vi "BotSpeakSerial_WriteRead1.vi"(4 "To Write":string, 5 "error In":errorcluster, 6 "Timeout":i32, 7 "Retries":i8, 8 "Address":string) -> (0 "error out":errorcluster, 1 "Reply":string, 2 "Reply EOF":string)   [LabVIEW 2012]
uses:
  <userlib>/botspeak/VIs/SubVIs/BotSpeak_Globals.vi
panel:
  out "iterations":i32
  out "Buffer":u32[](graph)
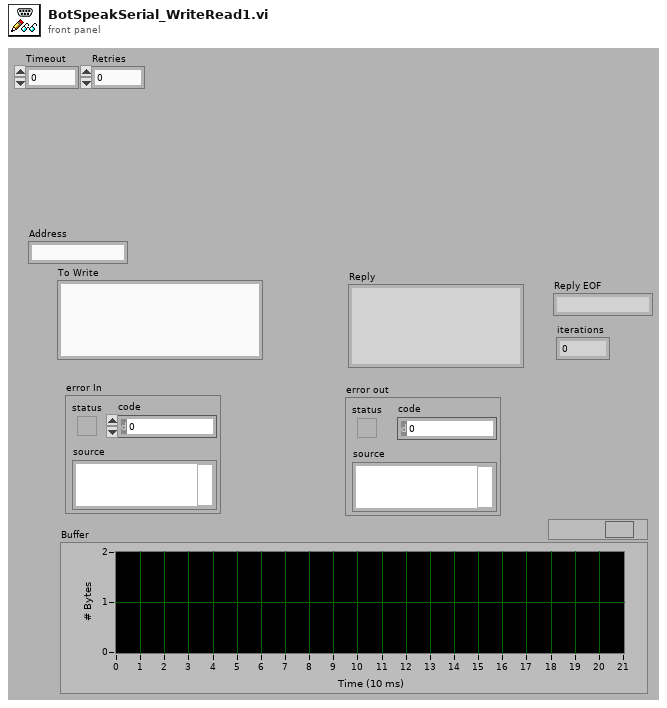
[diagram p1: front panel]
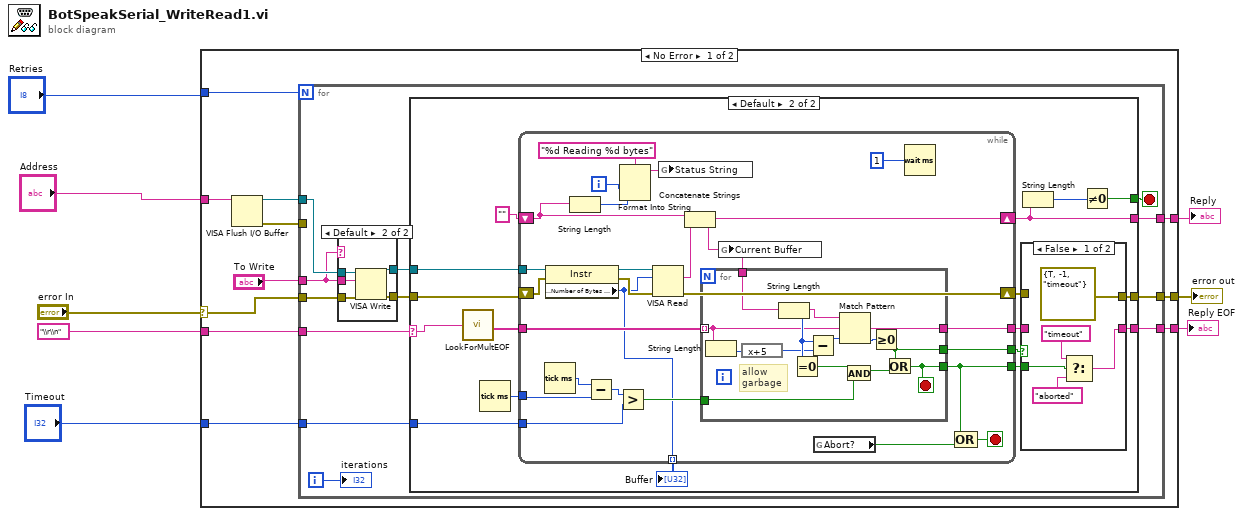
[diagram p0: block diagram]
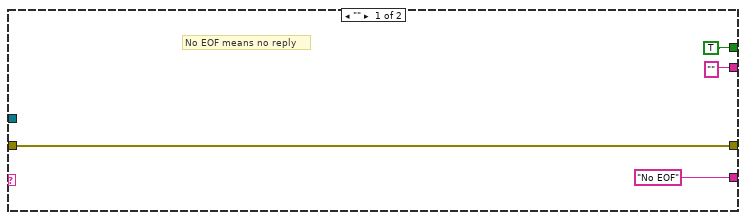
[diagram p3: hidden frame]
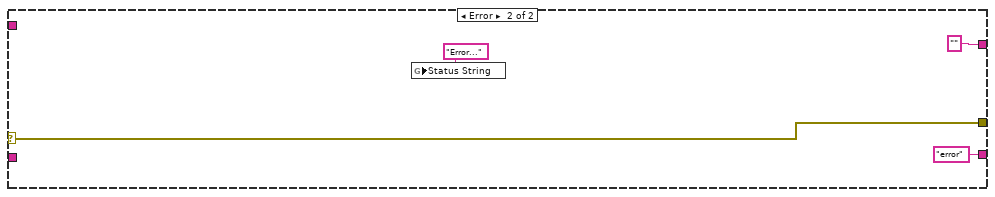
[diagram p5: hidden frame]
diagram:
  n1 = case shown="No Error" "error In" {
    selector: "error In" -> [w13 w105]
    tunnel: [w19 ""] -> w6
    tunnel: [w18 w105] -> w7
    tunnel: "Retries" -> [w17 _]
    tunnel: "Address" -> [w11 _]
    tunnel: "Timeout" -> [w16 _]
    tunnel: "\\r\\n" ("Reply EOF") -> [w14 _]
    tunnel: [w12 "error" ("Reply EOF")] -> w5
    frame No Error {
      n2 = VISA Flush I/O Buffer(VISA resource name=w11) -> (VISA resource name out=w9:refnum<visa-resource-name>, error out=w10:errorcluster)  [unwired: 2 in]
      n3 = for {
        N: w17 -> [_]
        tunnel: "To Write" -> [w21]
        tunnel: [w31] -> w19
        tunnel: [w27] -> w18
        tunnel: w13 -> [w30]
        tunnel: w16 -> [w25]
        tunnel: w14 -> [w24]
        tunnel: w9 -> [w23]
        tunnel: [w22] -> w12
        tunnel: w10 -> [_]
        i -> [w20]
        stop <- w26 stop-if-true
        n4 = case shown="Default" w21 {
          tunnel: w21 -> [_ w38]
          tunnel: w30 -> [w33 w37]
          tunnel: [w32 w36] -> w29
          tunnel: [w33 w35] -> w28
          tunnel: w23 -> [w32 w34]
          frame "" {
          }
          frame Default {
            n5 = VISA Write(VISA resource name=w34, write buffer=w38, error in (no error)=w37) -> (VISA resource name out=w36:refnum<visa-resource-name>, error out=w35:errorcluster)  [unwired: 1 out]
          }
        }
        n6 = case shown="Default" w24 {
          selector: w24 -> [_ w45]
          tunnel: ["" w55] -> w31
          tunnel: [w41 w44] -> w27
          tunnel: w29 -> [_ w58]
          tunnel: w28 -> [w41 w57]
          tunnel: [TRUE w47] -> w26
          tunnel: w25 -> [_ w53]
          tunnel: ["No EOF" ("Reply EOF") w49] -> w22
          frame "" {
            # "No EOF means no reply"
          }
          frame Default {
            n7 = call <userlib>:"LookForMultEOF.vi"("Reply EOF"=w45) -> ("Array"=w52:string[])
            n8 = Tick Count (ms)() -> (millisecond timer value=w56:u32)
            n9 = while {
              tunnel: w52 -> [w86]
              shift-right: [w91] -> w43
              shift-left: w57 -> [w90]
              shift-right: [w73] -> w55
              shift-left: "" -> [w76]
              tunnel: w58 -> [w85]
              tunnel: w56 -> [w80]
              tunnel: w53 -> [w71]
              tunnel: [w69] -> w51
              tunnel: [w70] -> w50
              tunnel: [w68] -> w48
              tunnel: [w67] -> w46 mode=indexing
              i -> [w78]
              stop <- w82 stop-if-true
              n10 = Tick Count (ms)() -> (millisecond timer value=w81:u32)
              n11 = property class="Instr"(reference=w85, error in=w90) -> (reference out=w89:refnum<visa-resource-name>, error out=w88:errorcluster, "Serial Settings:Number of Bytes at Serial Port"=w67:u32)
              n12 = String Length(string=w76) -> (length=w75:i32)
              n13 = Subtract(x=w81, y=w80) -> (x-y=w84:u32)
              n14 = Greater?(x=w84, y=w71) -> (0:w83:bool)
              n15 = Format Into String(format string="%d Reading %d bytes", w78, w75) -> (resulting string=w77:string)  [unwired: 2 in, 1 out]
              n16 = VISA Read(VISA resource name=w89, byte count=w67, error in (no error)=w88) -> (read buffer=w87:string, error out=w91:errorcluster)  [unwired: 2 out]
              n17 = global write "BotSpeak_Globals.vi" "Status String"(w77) -> ()
              n18 = Concatenate Strings(w76, w87) -> (w73:string)
              n19 = for {
                tunnel: w86 -> [w95] mode=indexing
                tunnel: w83 -> [w102]
                tunnel: w73 -> [w93]
                tunnel: [w96] -> w68
                tunnel: [w95] -> w70
                tunnel: [w94] -> w69
                stop <- w96 stop-if-true
                # "allow\ngarbage"
                n20 = String Length(string=w95) -> (length=w100:i32)
                n21 = expression code="x+5"(w100) -> (w92:i32)
                n22 = String Length(string=w93) -> (length=w98:i32)
                n23 = Equal To 0?(x=w98) -> (x = 0?=w101:bool)
                n24 = Subtract(x=w98, y=w92) -> (x-y=w99:i32)
                n25 = Match Pattern(string=w93, regular expression=w95, offset (0)=w99) -> (offset past match=w103:i32)  [unwired: 3 out]
                n26 = And(x=w101, y=w102) -> (x .and. y?=w97:bool)
                n27 = Greater Or Equal To 0?(x=w103) -> (x >= 0?=w94:bool)
                n28 = Or(x=w94, y=w97) -> (x .or. y?=w96:bool)
              }
              n29 = global write "BotSpeak_Globals.vi" "Current Buffer"(w73) -> ()
              n30 = global read "BotSpeak_Globals.vi" "Abort?"() -> (w72:bool)
              n31 = Wait (ms)(milliseconds to wait=u32 1) -> ()  [unwired: 1 out]
              n32 = Compound Arithmetic op=OR(w68, w72) -> (w82:bool)
            }
            "Buffer" <- w46
            n33 = case shown="False" w51 {
              tunnel: w50 -> [_ w66]
              tunnel: [w61 w66] -> w49
              tunnel: w48 -> [w63 _]
              tunnel: [errorcluster {"status"=TRUE, "code"=-1, "source"="timeout"} ("error out") w65] -> w44
              tunnel: w43 -> [_ w65]
              frame False {
                n34 = Select(t="timeout" ("Reply EOF"), s=w63, f="aborted" ("Reply EOF")) -> (s? t:f=w61:string)
              }
              frame True {
              }
            }
            n35 = String Length(string=w55) -> (length=w54:i32)
            n36 = Not Equal To 0?(x=w54) -> (x != 0?=w47:bool)
          }
        }
        "iterations" <- w20
      }
    }
    frame Error {
      n37 = global write "BotSpeak_Globals.vi" "Status String"("Error..." ("Status String")) -> ()
    }
  }
  "error out" <- w7
  "Reply" <- w6
  "Reply EOF" <- w5
